vi "Initialize Workspace Control Refs.vi"(7 "T = PID":bool, 9 "State Variables in":T1={"UI.Refs"={"Chart"=refnum, "Manual Value"=refnum, "Manual Output"=refnum, "Revert"=refnum, "Apply"=refnum}, "Addon.GUID"="", "Addon.Name"="", "Addon.Type"=enum."Industrial", "Data.UDPEngineQueue"=refnum, "Data.Found?"=FALSE, "Data.UDPChannels"=[], "Data.PreviousValues"=[], "Data.SlowChannels"=[], "Data.PendingChange?"=FALSE, "CachedData.UserEvent"=refnum, "CachedData.Data"={"Path"=""}, "Workspace.Connected?"=FALSE, "NIVS.SysDef"=refnum, "NIVS.WorkspaceManager"=refnum, "NIVS.UserEventRefs"={"Event Registration Refnum"=refnum, "SystemChangeEventRef"=refnum}, "NIVS.SystemStateRefs"={"CustDatRef"=refnum, "EvtRef"=refnum, "Target State User Event"=refnum}, "NIVS.LaunchRef"=refnum, "Setpoint Range"={"Min"=0.0, "Max"=0.0}, "Output Range"={"Min"=0.0, "Max"=0.0}}, 10 "Item.Data":T7, 11 "NIVS.Gateway IP Address":string) -> (0 "error out":errorcluster, 3 "State Variables out":T1={"UI.Refs"={"Chart"=refnum, "Manual Value"=refnum, "Manual Output"=refnum, "Revert"=refnum, "Apply"=refnum}, "Addon.GUID"="", "Addon.Name"="", "Addon.Type"=enum."Industrial", "Data.UDPEngineQueue"=refnum, "Data.Found?"=FALSE, "Data.UDPChannels"=[], "Data.PreviousValues"=[], "Data.SlowChannels"=[], "Data.PendingChange?"=FALSE, "CachedData.UserEvent"=refnum, "CachedData.Data"={"Path"=""}, "Workspace.Connected?"=FALSE, "NIVS.SysDef"=refnum, "NIVS.WorkspaceManager"=refnum, "NIVS.UserEventRefs"={"Event Registration Refnum"=refnum, "SystemChangeEventRef"=refnum}, "NIVS.SystemStateRefs"={"CustDatRef"=refnum, "EvtRef"=refnum, "Target State User Event"=refnum}, "NIVS.LaunchRef"=refnum, "Setpoint Range"={"Min"=0.0, "Max"=0.0}, "Output Range"={"Min"=0.0, "Max"=0.0}})   [LabVIEW 2019, in "Control Workspace Object.lvlib"]
uses:
  Control Workspace Object.lvlib
  <vilib>/NI VeriStand/Display Template Support/DisplayTemplateSupport.llb/cluster_Screen Item Settings.ctl
  <vilib>/NI VeriStand/Display Template Support/DisplayTemplateSupport.llb/cluster_Graph Scale Settings.ctl
  <vilib>/NI VeriStand/Display Template Support/DisplayTemplateSupport.llb/cluster_Graph Plot Settings.ctl
  Shared/Types/Workspace Object State Variables.ctl
  Shared/Types/UI.Refs.ctl
  Shared/Types/UDP Streaming Command Cluster.ctl
  Shared/Types/UDP Streaming State.ctl
  <vilib>/NI VeriStand/Display Template Support/DisplayTemplateSupport.llb/enum_Display Template Handler Minimal To Workspace.ctl
  Shared/Types/Workspace Object Cached Settings.ctl
  NationalInstruments.VeriStand.SystemStorage
  <vilib>/NI VeriStand/Execution/Workspace/WorkspaceAPI.ctl
  NationalInstruments.VeriStand.ClientAPI
  <vilib>/NI VeriStand/Display Template Support/DisplayTemplateSupport.llb/enum_Display Template Handler Minimal To Widget Msg.ctl
  <vilib>/NI VeriStand/Execution/Workspace/SystemStateRegEventRef.ctl
  <vilib>/NI VeriStand/Execution/Workspace/Target State Info.ctl
  <vilib>/NI VeriStand/Execution/Workspace/Target State.ctl
  <vilib>/NI VeriStand/Execution/Workspace/SystemStateEventRef.ctl
  Shared/Constants.vi
  <vilib>/NI VeriStand/Execution/Workspace/NI_VS Workspace ExecutionAPI.lvlib
  Shared/Control Addon Shared.lvlib
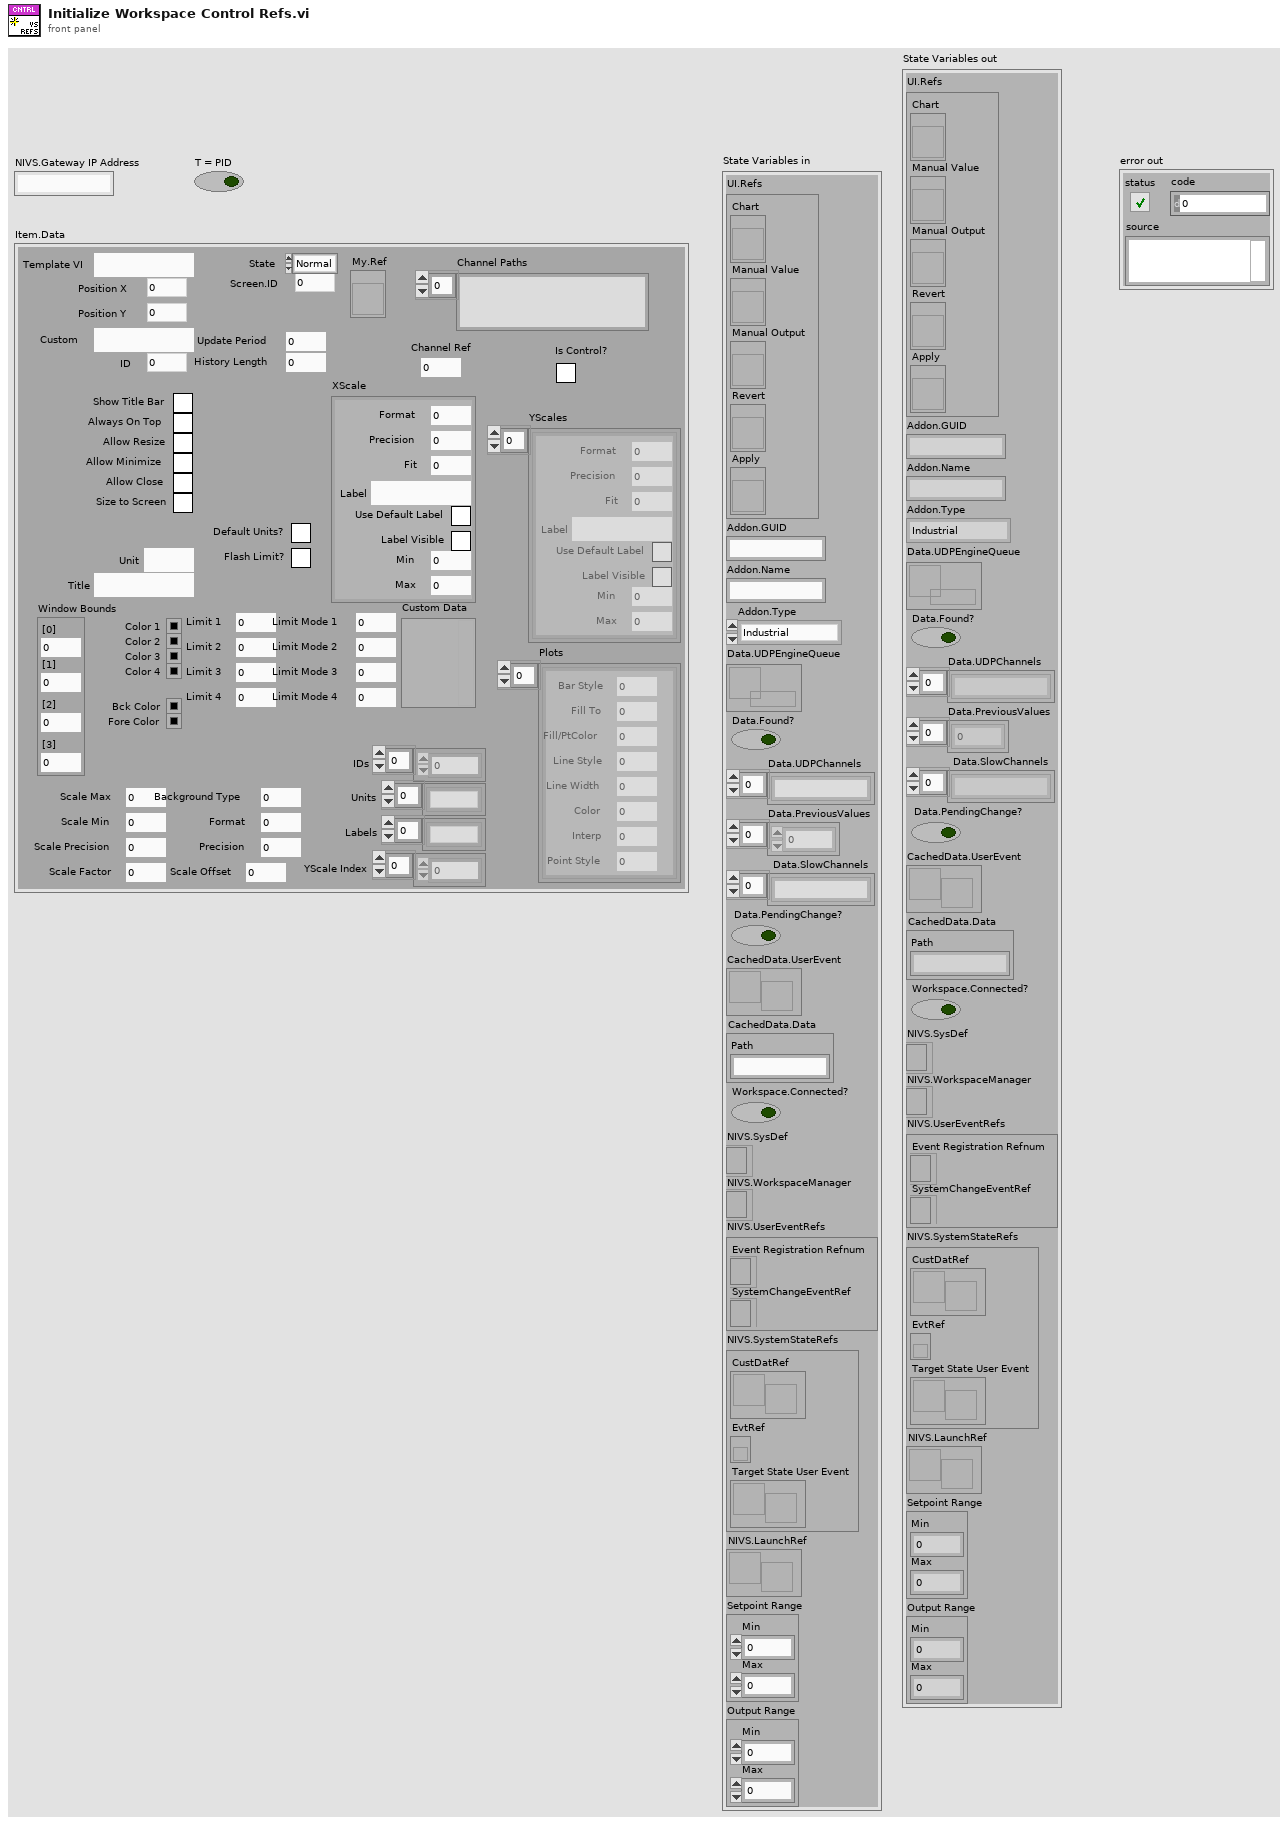
[diagram p1: front panel]
types:
  T1 = typedef "Control Addon Shared.lvlib/Workspace Object State Variables.ctl" = cluster{"UI.Refs":T2, "Addon.GUID":string, "Addon.Name":string, "Addon.Type":enum16{"PID", "Industrial"}, "Data.UDPEngineQueue":refnum<queue>, "Data.Found?":bool, "Data.UDPChannels":string[], "Data.PreviousValues":dbl[], "Data.SlowChannels":string[], "Data.PendingChange?":bool, "CachedData.UserEvent":refnum<user-event>, "CachedData.Data":T3, "Workspace.Connected?":bool, "NIVS.SysDef":refnum<k24>, "NIVS.WorkspaceManager":T4, "NIVS.UserEventRefs":cluster{"Event Registration Refnum":refnum<event-registration>, "SystemChangeEventRef":T5}, "NIVS.SystemStateRefs":T6, "NIVS.LaunchRef":refnum<user-event>, "Setpoint Range":cluster{"Min":dbl, "Max":dbl}, "Output Range":cluster{"Min":dbl, "Max":dbl}}
  T2 = typedef "Control Addon Shared.lvlib/UI.Refs.ctl" = cluster{"Chart":refnum<vi>, "Manual Value":refnum<vi>, "Manual Output":refnum<vi>, "Revert":refnum<vi>, "Apply":refnum<vi>}
  T3 = typedef "Control Addon Shared.lvlib/Workspace Object Cached Settings.ctl" = cluster{"Path":string}
  T4 = typedef "NI_VS Workspace ExecutionAPI.lvlib/WorkspaceAPI.ctl" = refnum<k24>
  T5 = typedef "NI_VS Workspace ExecutionAPI.lvlib/SystemStateRegEventRef.ctl" = refnum<event-registration>
  T6 = typedef "NI_VS Workspace ExecutionAPI.lvlib/SystemStateEventRef.ctl" = cluster{"CustDatRef":refnum<user-event>, "EvtRef":refnum<k27>, "Target State User Event":refnum<user-event>}
  T7 = typedef "cluster_Screen Item Settings.ctl" = cluster{"Template VI":string, "Position X":i32, "Position Y":i32, "Custom":string, "Show Title Bar":bool, "ID":i32, "Always On Top":bool, "Allow Resize":bool, "Allow Minimize":bool, "Allow Close":bool, "Size to Screen":bool, "Screen.ID":i32, "State":enum16{"Normal", "New"}, "Title":string, "Window Bounds":cluster{"[0]":i16, "[1]":i16, "[2]":i16, "[3]":i16}, "Channel Ref":u64, "Unit":string, "Default Units?":bool, "Flash Limit?":bool, "Color 1":u32, "Color 2":u32, "Color 3":u32, "Color 4":u32, "Bck Color":u32, "Fore Color":u32, "Limit 1":dbl, "Limit 2":dbl, "Limit 3":dbl, "Limit 4":dbl, "Limit Mode 1":i32, "Limit Mode 2":i32, "Limit Mode 3":i32, "Limit Mode 4":i32, "Scale Precision":i32, "Scale Min":dbl, "Scale Max":dbl, "Format":i32, "Precision":i32, "Background Type":i32, "IDs":i32[], "Units":string[], "Labels":string[], "Scale Factor":dbl, "Scale Offset":dbl, "YScale Index":u32[], "XScale":T8, "YScales":T8[], "Plots":T9[], "Update Period":dbl, "History Length":dbl, "My.Ref":refnum<vi>, "Is Control?":bool, "Channel Paths":string[], "Custom Data":variant}
  T8 = typedef "cluster_Graph Scale Settings.ctl" = cluster{"Format":u8, "Precision":u8, "Fit":u8, "Label":string, "Use Default Label":bool, "Label Visible":bool, "Min":dbl, "Max":dbl}
  T9 = typedef "cluster_Graph Plot Settings.ctl" = cluster{"Bar Style":u8, "Fill To":i16, "Fill/PtColor":u32, "Line Style":u8, "Line Width":u8, "Color":u32, "Interp":u8, "Point Style":u8}
  T10 = typedef "Control Addon Shared.lvlib/UDP Streaming Command Cluster.ctl" = cluster{"Action":T11, "Channels":string[]}
  T11 = typedef "Control Addon Shared.lvlib/UDP Streaming State.ctl" = enum8{"Idle", "Start Acq", "Run", "Stop Acq", "Exit"}
  T12 = cluster{"Event Registration Refnum":refnum<event-registration>, "SystemChangeEventRef":T5}
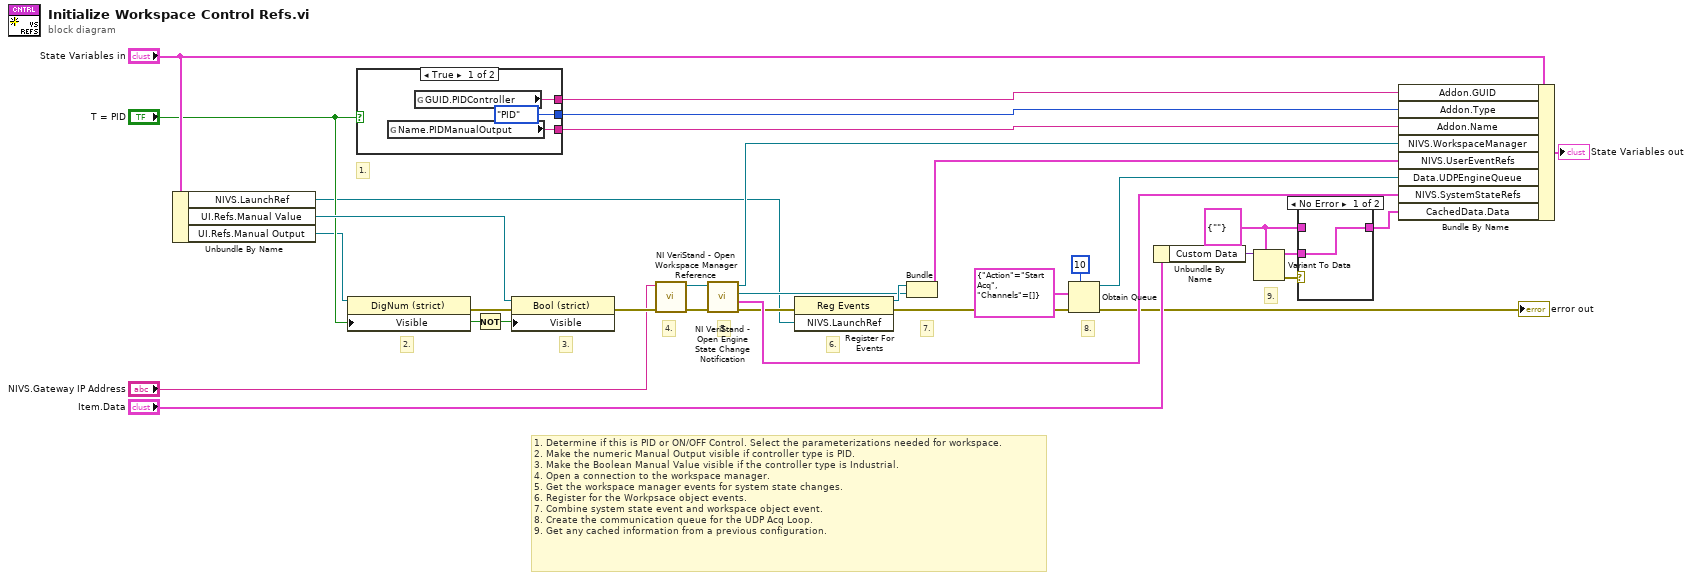
[diagram p0: block diagram]
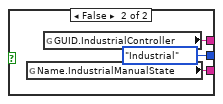
[diagram p2: hidden frame]
diagram:
  w15 = T3 {"Path"=""}
  # "1. Determine if this is PID or ON/OFF Control. Select the parameterizations needed for workspace.\n2. Make the numeric Manual Output visible if controller type is PID.\n3. Make the Boolean Manual Value visible if the controller type is Industrial.\n4. Open a connection to the workspace manager.\n5. Get the workspace manager events for system state changes.\n6. Register for the Workpsace object events.\n7. Combine system state event and workspace object event.\n8. Create the communication queue for the UDP Acq Loop.\n9. Get any cached information from a previous configuration."
  # "9."
  # "8."
  # "7."
  # "6."
  # "5."
  # "4."
  # "3."
  # "2."
  # "1."
  n1 = Unbundle By Name("State Variables in") -> ("NIVS.LaunchRef"=w3:refnum<user-event>, "UI.Refs.Manual Value"=w27:refnum<vi>, "UI.Refs.Manual Output"=w25:refnum<vi>)
  n2 = property class="DigNum (strict)"(reference=w25, "Visible"="T = PID") -> (error out=w29:errorcluster)  [unwired: 1 in, 1 out]
  n3 = case shown="True" "T = PID" {
    tunnel: [w35 w38] -> w20
    tunnel: [w33 w37] -> w18
    tunnel: [enum16{"PID", "Industrial"}."PID" ("Type") enum16{"PID", "Industrial"}."Industrial" ("Type")] -> w19
    frame True {
      n4 = global read "Constants.vi" "Name.PIDManualOutput"() -> (w33:string)
      n5 = global read "Constants.vi" "GUID.PIDController"() -> (w35:string)
    }
    frame False {
      n6 = global read "Constants.vi" "Name.IndustrialManualState"() -> (w37:string)
      n7 = global read "Constants.vi" "GUID.IndustrialController"() -> (w38:string)
    }
  }
  n8 = Not(x="T = PID") -> (.not. x?=w28:bool)
  n9 = property class="Bool (strict)"(reference=w27, error in=w29, "Visible"=w28) -> (error out=w30:errorcluster)  [unwired: 1 out]
  n10 = call <vilib>:"NI VeriStand - Open Workspace Manager Reference.vi"("error in (no error)"=w30, "Gateway IP Address (\"\": localhost)"="NIVS.Gateway IP Address") -> ("error out"=w9:errorcluster, "WorkspaceManager"=w23:T4)  [unwired: 8 in]
  n11 = call <vilib>:"NI VeriStand - Open Engine State Change Notification.vi"("error in (no error)"=w9, "WorkspaceManager in"=w23) -> ("error out"=w5:errorcluster, "SystemStateRefs"=w22:T6, "SystemChangeEventRef"=w10:T5, "WorkspaceManager out"=w6:T4)  [unwired: 6 in]
  n12 = register-events(error in=w5, w3) -> (reference out=w11:refnum<event-registration>, error out=w4:errorcluster)  [unwired: 1 in]
  n13 = Bundle("Event Registration Refnum"=w11, "SystemChangeEventRef"=w10) -> (w21:T12)  [unwired: 1 in]
  n14 = Obtain Queue(max queue size (-1, unlimited)=10, element data type=T10 {"Action"=enum."Start Acq", "Channels"=[]}, error in (no error)=w4) -> (queue out=w2:refnum<queue>, error out=→"error out":errorcluster)  [unwired: 2 in, 1 out]
  n15 = Unbundle By Name("Item.Data") -> ("Custom Data"=w12:variant)
  n16 = Variant To Data(type=w15, Variant=w12) -> (data=w14:T3, error out=w13:errorcluster)  [unwired: 1 in]
  n17 = case shown="No Error" w13 {
    tunnel: w14 -> [w39 _]
    tunnel: [w39 w40] -> w1
    tunnel: w15 -> [_ w40]
    frame No Error {
    }
    frame Error {
    }
  }
  n18 = Bundle By Name(cluster="State Variables in", "Addon.GUID"=w20, "Addon.Type"=w19, "Addon.Name"=w18, "NIVS.WorkspaceManager"=w6, "NIVS.UserEventRefs"=w21, "Data.UDPEngineQueue"=w2, "NIVS.SystemStateRefs"=w22, "CachedData.Data"=w1) -> (→"State Variables out":T1)
